vi "Popup - Tools.vi"() -> (2 "Output Tools":T1, 3 "Cancelled?":bool)   [LabVIEW 2020]
panel:
  in  "Cancel Button":bool
  in  "Add Button":bool
  in  "Serial No.":string
  in  "Description":string
  in  "ID":string
  in  "Type":string
  # "ADD TOOLS"
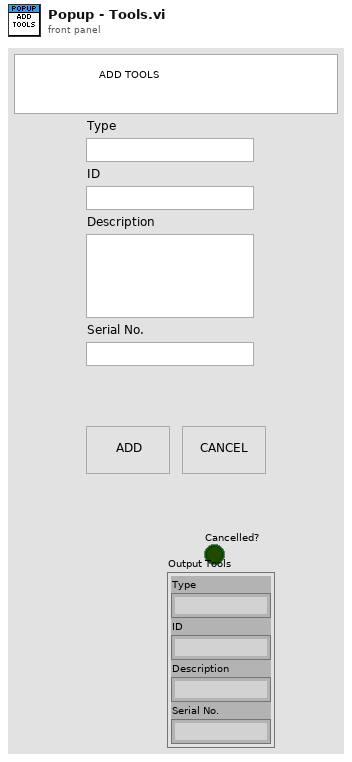
[diagram p1: front panel]
types:
  T1 = cluster{"Type":string, "ID":string, "Description":string, "Serial No.":string}
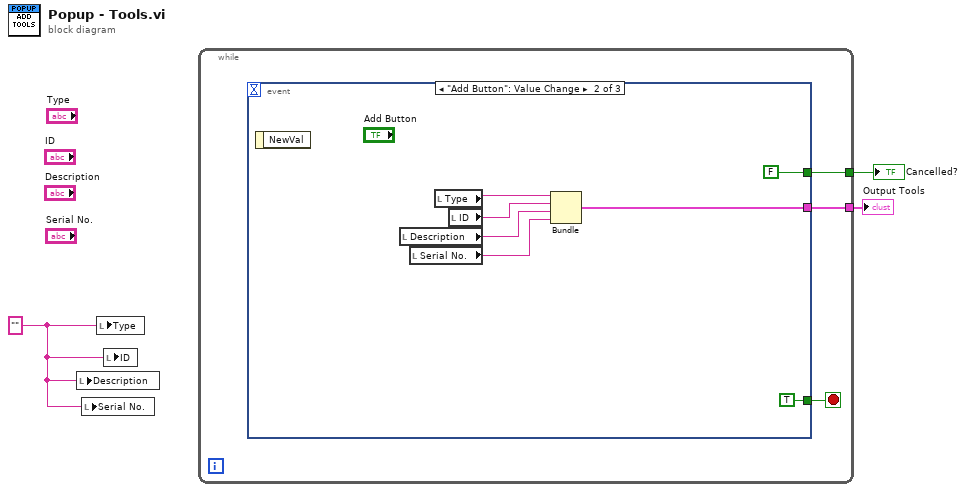
[diagram p0: block diagram]
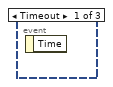
[diagram p2: hidden frame]
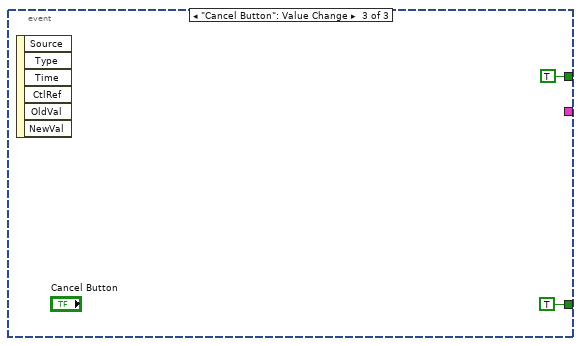
[diagram p3: hidden frame]
diagram:
  w2 = "" ("Type")
  n1 = local write "Description"(w2) -> ()
  n2 = local write "Serial No."(w2) -> ()
  n3 = local write "Type"(w2) -> ()
  n4 = local write "ID"(w2) -> ()
  n5 = while {
    tunnel: [w6] -> w1
    tunnel: [w5] -> w3
    stop <- w4 stop-if-true
    n6 = event shown="[1] \"Add Button\": Value Change" {
      selector: _ -> [_ _ _]
      dyn-events: _ -> [_ _ _]
      timeout: _ -> [_ _ _]
      tunnel: [_ w9 _] -> w6
      tunnel: [_ FALSE TRUE] -> w5
      tunnel: [_ TRUE TRUE] -> w4
      event Timeout {
        n7 = event-data() -> ()  [unwired: 1 in, 1 out]
      }
      event "Add Button": Value Change {
        n8 = event-data() -> ()  [unwired: 1 in, 1 out]
        n9 = local read "Description"() -> (w11:string)
        n10 = local read "Serial No."() -> (w10:string)
        n11 = local read "Type"() -> (w13:string)
        n12 = local read "ID"() -> (w12:string)
        n13 = Bundle("Type"=w13, "ID"=w12, "Description"=w11, "Serial No."=w10) -> (w9:T1)  [unwired: 1 in]
      }
      event "Cancel Button": Value Change {
        n14 = event-data() -> ()  [unwired: 1 in, 6 out]
      }
    }
  }
  "Cancelled?" <- w3
  "Output Tools" <- w1
